vi "PopUp.vi"(8 "error in (no error)":errorcluster, 10 "String":string, 11 "First Actor in":refnum<class "First Actor.lvclass">) -> (0 "error out":errorcluster, 3 "First Actor out":refnum<class "First Actor.lvclass">)   [LabVIEW 2020, in "First Actor.lvlib" / "First Actor.lvclass"]
uses:
  First Actor.lvclass
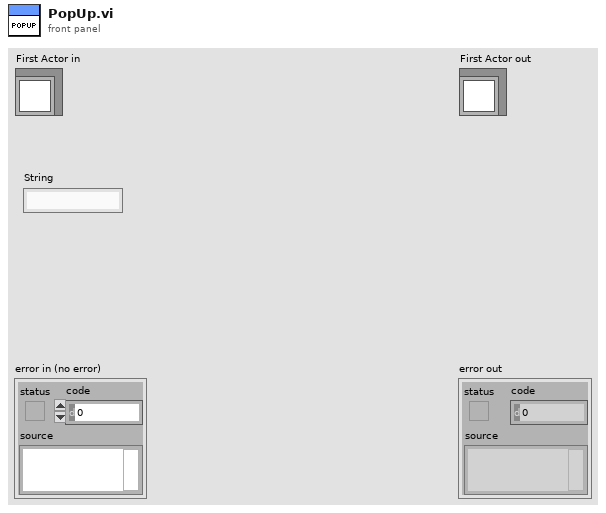
[diagram p1: front panel]
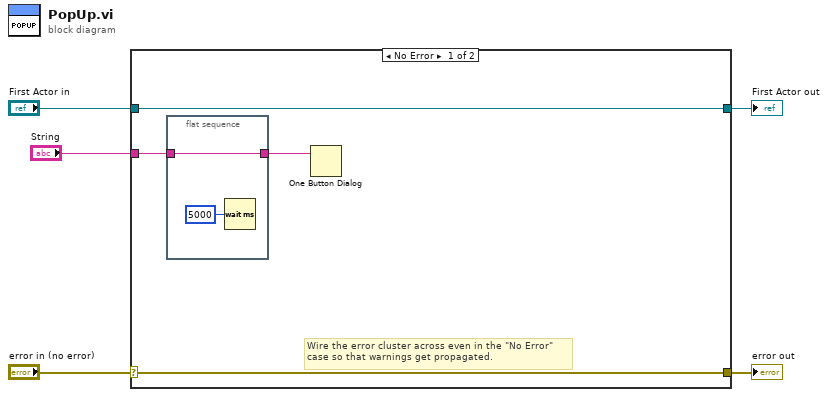
[diagram p0: block diagram]
diagram:
  n1 = case shown="No Error" "error in (no error)" {
    selector: "error in (no error)" -> [w8 w13]
    tunnel: [w8 w13] -> w4
    tunnel: [w9 w12] -> w2
    tunnel: "First Actor in" -> [w9 w12]
    tunnel: "String" -> [w7 _]
    frame No Error {
      # "Wire the error cluster across even in the \"No Error\"\ncase so that warnings get propagated."
      n2 = flat-sequence {
        tunnel: w7 -> [w11]
        tunnel: [w11] -> w6
        frame #0 {
          n3 = Wait (ms)(milliseconds to wait=u32 5000) -> ()  [unwired: 1 out]
        }
      }
      n4 = One Button Dialog(message=w6) -> ()  [unwired: 1 in, 1 out]
    }
    frame Error {
    }
  }
  "error out" <- w4
  "First Actor out" <- w2
